vi "PRL PMU Status.vi"(8 "error in (no error)":errorcluster) -> (0 "error out":errorcluster, 3 "PMU Status":T1(array[cluster]))   [LabVIEW 2013, in "PMU Recorder Light.lvlib"]
uses:
  PMU Recorder Light.lvlib
panel:
  # "INPUT"
  # "INTERMEDIATE"
  # "OUTPUT"
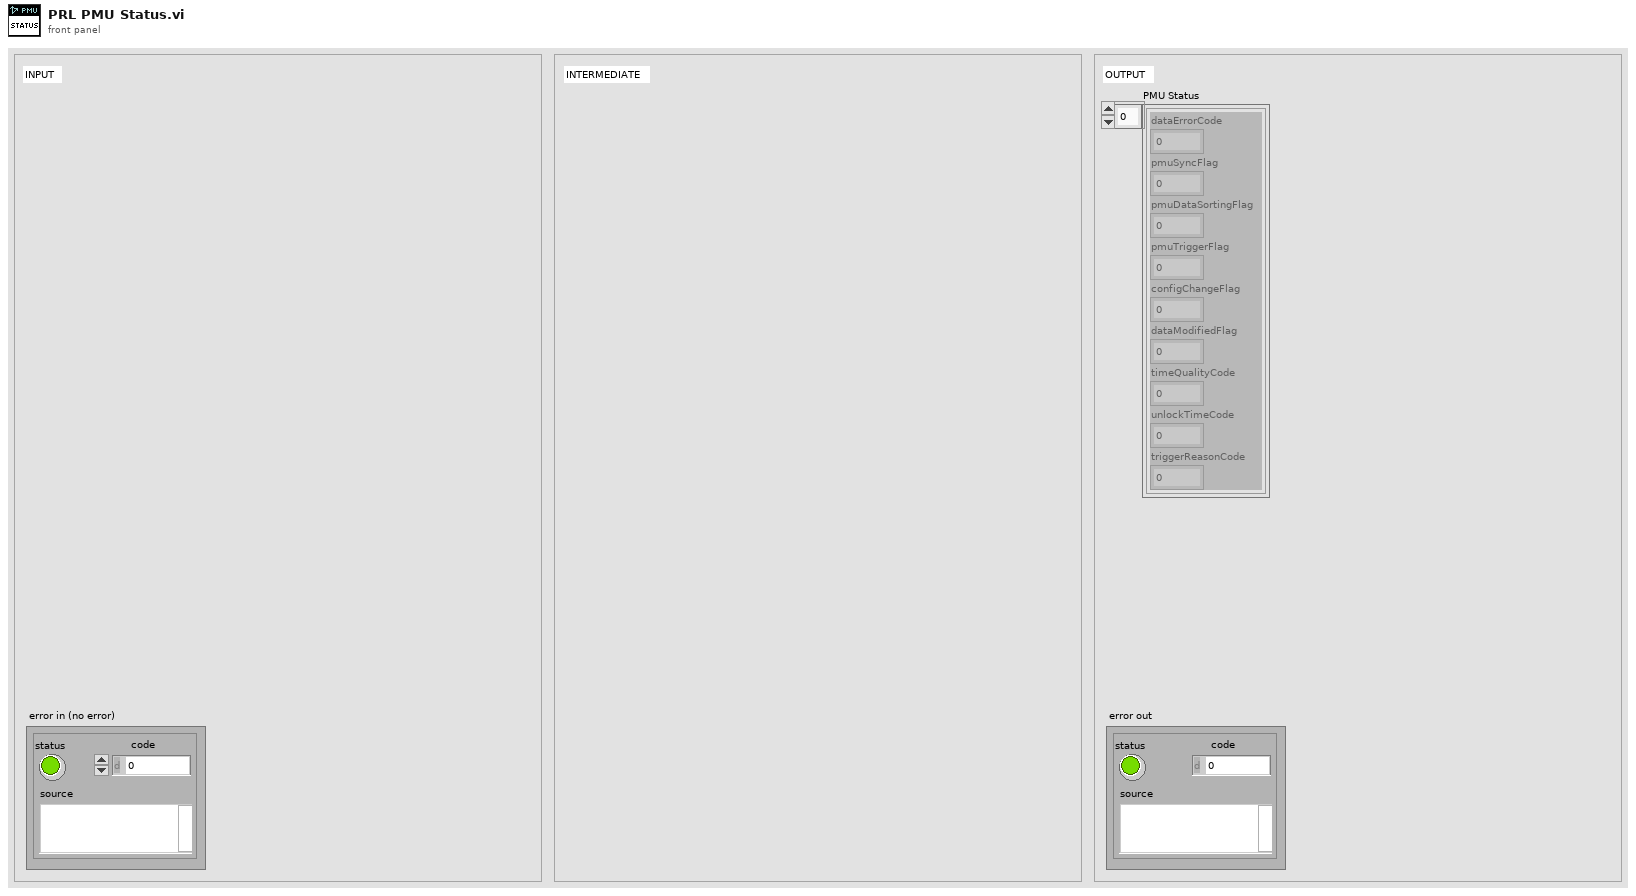
[diagram p1: front panel]
types:
  T1 = cluster{"dataErrorCode":u8, "pmuSyncFlag":u8, "pmuDataSortingFlag":u8, "pmuTriggerFlag":u8, "configChangeFlag":u8, "dataModifiedFlag":u8, "timeQualityCode":u8, "unlockTimeCode":u8, "triggerReasonCode":u8}[]
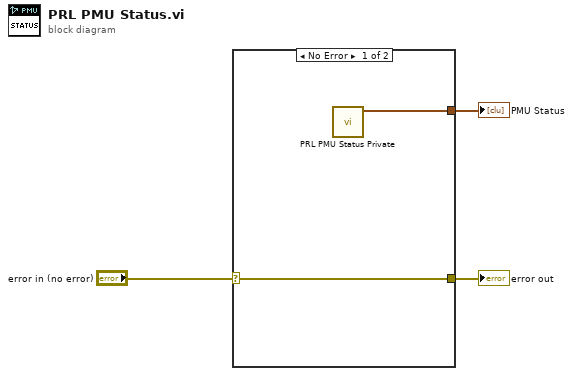
[diagram p0: block diagram]
diagram:
  n1 = case shown="No Error" "error in (no error)" {
    selector: "error in (no error)" -> [w4 w6]
    tunnel: [w5 _] -> w3
    tunnel: [w4 w6] -> w1
    frame No Error {
      n2 = call "PRL PMU Status Private.vi"() -> ("PMU Status Out"=w5:T1)  [unwired: 11 in]
    }
    frame Error {
    }
  }
  "PMU Status" <- w3
  "error out" <- w1
